vi "FunctionGraph.vi"() -> ()   [LabVIEW 2014]
panel:
  in  "xmax":dbl=5.0
  in  "xmin":dbl=-5.0
  in  "Update":bool
  in  "stop":bool
  in  "w":dbl=1.0
  in  "A":dbl=1.0
  in  "Function":enum16{"A*sin(w*x)", "A*cos(w*x)", "A*tan(w*x)"}(ring)
  out "Function XY Graph":cluster{"Ramp Pattern":dbl[], dbl[]}(graph)
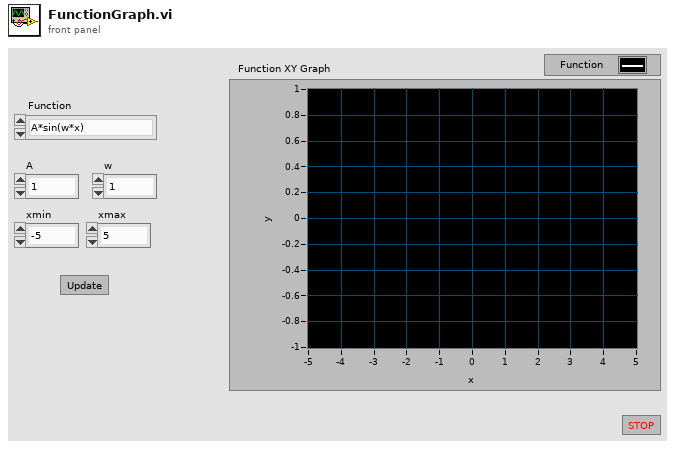
[diagram p1: front panel]
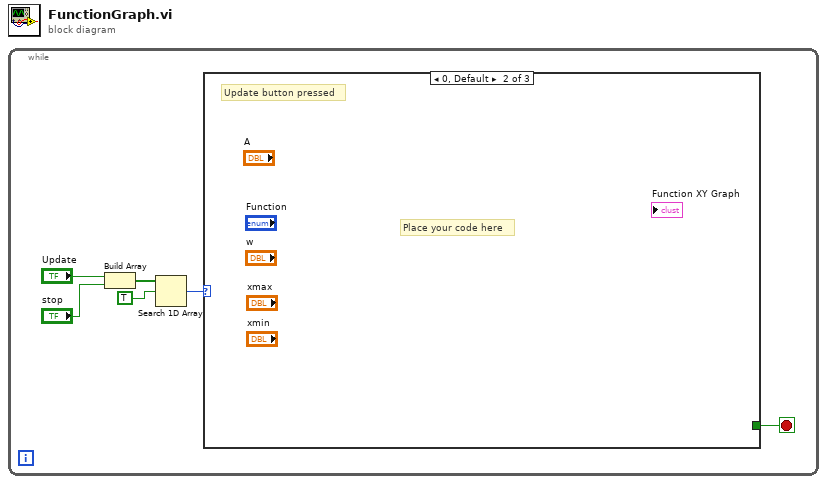
[diagram p0: block diagram]
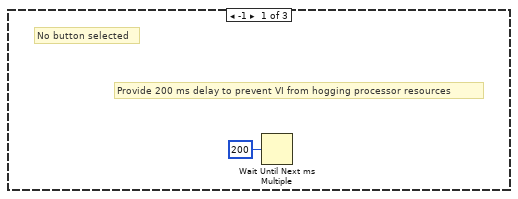
[diagram p2: hidden frame]
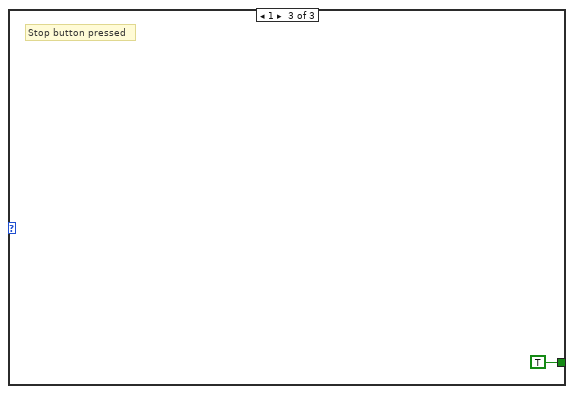
[diagram p3: hidden frame]
diagram:
  n1 = while {
    stop <- w1 stop-if-true
    n2 = Build Array("Update", "stop") -> (w4:bool[])
    n3 = Search 1D Array(1D array=w4, element=TRUE) -> (index of element=w2:i32)  [unwired: 1 in]
    n4 = case shown="0, Default" w2 {
      tunnel: [_ _ TRUE] -> w1
      frame -1 {
        # "Provide 200 ms delay to prevent VI from hogging processor resources"
        # "No button selected"
        n5 = Wait Until Next ms Multiple(millisecond multiple=u32 200) -> ()  [unwired: 1 out]
      }
      frame 0, Default {
        # "Place your code here"
        # "Update button pressed"
      }
      frame 1 {
        # "Stop button pressed"
      }
    }
  }
